vi "Ctor.vi"(8 "error in (no error)":errorcluster, 11 "Game Config Panel in":refnum<class "Game Config Panel.lvclass">) -> (0 "error out":errorcluster, 3 "Game Config Panel out":refnum<class "Game Config Panel.lvclass">)   [LabVIEW 2020, in "SB App.lvlib" / "Game Config Panel.lvclass"]
uses:
  Game Config Panel.lvclass
  Add Team Data.ctl
  SquareBattle/Team/Team.lvclass
  Start Position Data.ctl
  SquareBattle/Team ID.ctl
  SquareBattle/Position.ctl
  Game Config Panel.lvclass/Game Config Panel.ctl
  <vilib>/IlluminatedG/IG OOPanel/OOPanel/Panel/Panel.lvclass
  SquareBattle/SquareBattle.lvlib
  SB App.lvlib
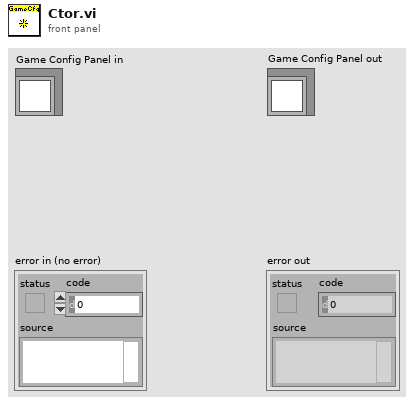
[diagram p1: front panel]
types:
  T1 = typedef "SquareBattle.lvlib/Team ID.ctl" = u32
  T2 = typedef "SB App.lvlib/Start Position Data.ctl" = cluster{"Team ID":T1, "Position":T3}
  T3 = typedef "SquareBattle.lvlib/Position.ctl" = cluster{"Row":i32, "Col":i32}
  T4 = typedef "SB App.lvlib/Game Config Panel.lvclass/Add Team Data.ctl" = cluster{"Team":refnum<class "Team.lvclass">}
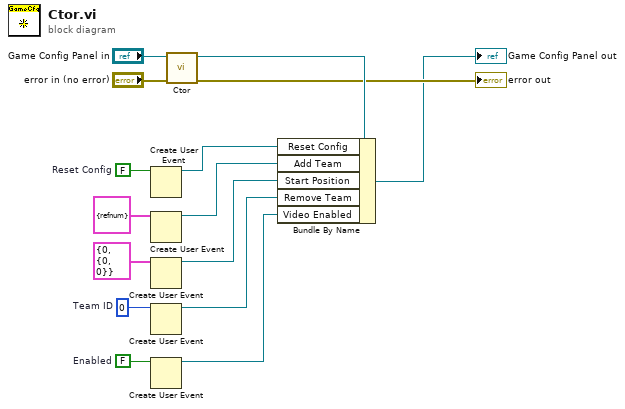
[diagram p0: block diagram]
diagram:
  w2 = FALSE  # Enabled
  w4 = T1 0  # Team ID
  w10 = FALSE  # Reset Config
  n1 = Create User Event(user event datatype=w10) -> (user event=w9:refnum<user-event>)  [unwired: 1 in, 1 out]
  n2 = Create User Event(user event datatype=T4 {"Team"=refnum} ("Add Team Data")) -> (user event=w7:refnum<user-event>)  [unwired: 1 in, 1 out]
  n3 = Create User Event(user event datatype=T2 {"Team ID"=0, "Position"={"Row"=0, "Col"=0}} ("Start Position Data")) -> (user event=w5:refnum<user-event>)  [unwired: 1 in, 1 out]
  n4 = Create User Event(user event datatype=w4) -> (user event=w3:refnum<user-event>)  [unwired: 1 in, 1 out]
  n5 = Create User Event(user event datatype=w2) -> (user event=w1:refnum<user-event>)  [unwired: 1 in, 1 out]
  n6 = call-parent "Ctor.vi"("error in (no error)"="error in (no error)", "Panel in"="Game Config Panel in") -> ("error out"=→"error out":errorcluster, "Panel out"=w13:refnum<class "Game Config Panel.lvclass">)  [unwired: 8 in]
  n7 = Bundle By Name(cluster=w13, "Reset Config"=w9, "Add Team"=w7, "Start Position"=w5, "Remove Team"=w3, "Video Enabled"=w1) -> (→"Game Config Panel out":refnum<class "Game Config Panel.lvclass">)
